vi "ScopeDAQ.vi"() -> ()   [LabVIEW 2021]
uses:
  <instrlib>/Tektronix TDS 200 1000 2000 Series/Public/Configure/Configure Trigger (Edge).vi
  <instrlib>/Tektronix TDS 200 1000 2000 Series/Tektronix TDS 200 1000 2000 Series.lvlib
panel:
  in  "Signal Source (Channel)":u16(ring) items=["Channel 1", "Channel 2", "Channel 3", "Channel 4", "Math", "Reference A", "Reference B", "Reference C", "Reference D"]
  in  "Position (0.0 s)":dbl
  out "Waveform Graph":waveform(dbl)(graph)={"t0"=timestamp(-2.500000000016378e-06 s since 1904-01-01), "dt"=2e-09, "Y"=array[2500 elements]}
  in  "Trigger Level (V)":dbl=-0.368
  in  "Vertical Range (V/div)":dbl=0.5
  in  "Timebase (s/div)":dbl=5e-07
  in  "Vertical Coupling":i32(ring) items=["AC", "DC", "Ground"]
  in  "Serial Configuration":T1={"Baud Rate"=19200, "Parity"=0, "Stop Bits"=10, "Flow Control"=2} {"Flow Control" items=["None", "XON/XOFF", "RTS/CTS", "XON/XOFF & RTS/CTS", "DTR/DSR", "XON/XOFF & DTR/DSR"]; "Stop Bits" items=["1.0"=10, "1.5"=15, "2.0"=20]; "Parity" items=["None", "Odd", "Even", "Mark", "Space"]; "Baud Rate" items=["300"=300, "600"=600, "1200"=1200, "2400"=2400, "4800"=4800, "9600"=9600, "19200"=19200]}
  in  "Trigger Source (Channel)":u16(ring) items=["Channel 1", "Channel 2", "Channel 3", "Channel 4", "Math", "Reference A", "Reference B", "Reference C", "Reference D"]
  in  "stop":bool
  in  "Probe Attenuation":dbl=1.0
  in  "VISA resource name":refnum<visa-resource-name>="USB0::0x0699::0x0369::C057527::INSTR"
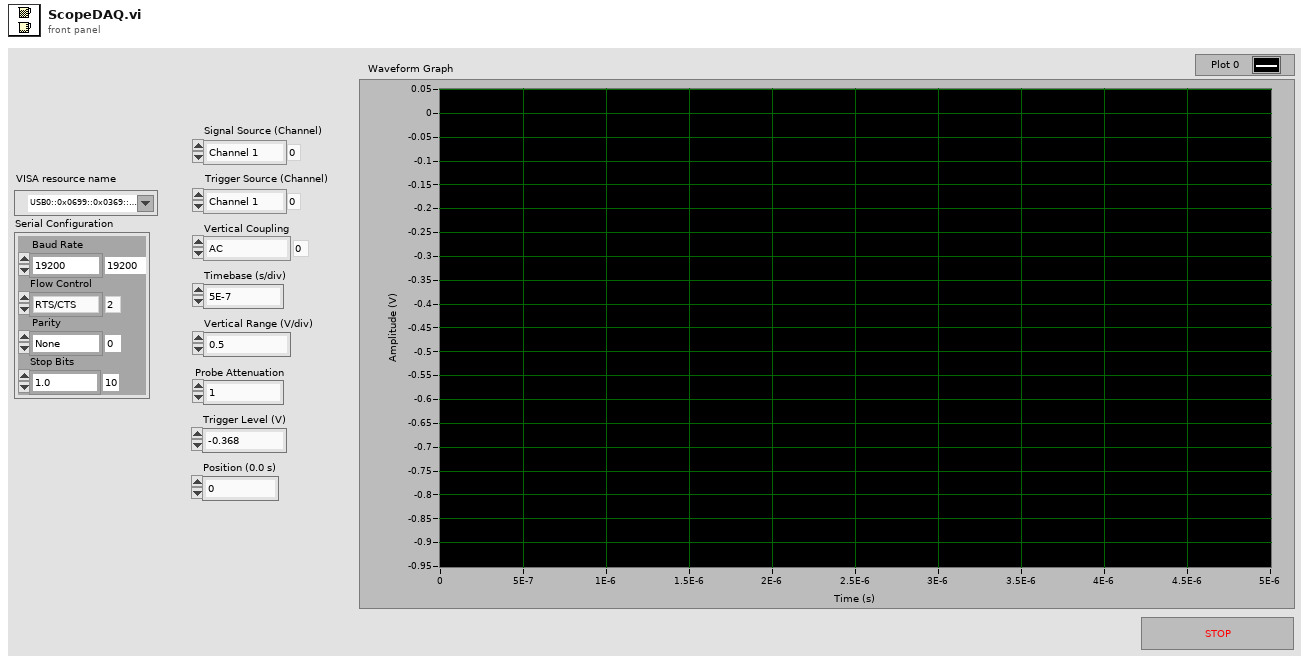
[diagram p1: front panel]
types:
  T1 = cluster{"Baud Rate":u32, "Parity":u16, "Stop Bits":u16, "Flow Control":u16}
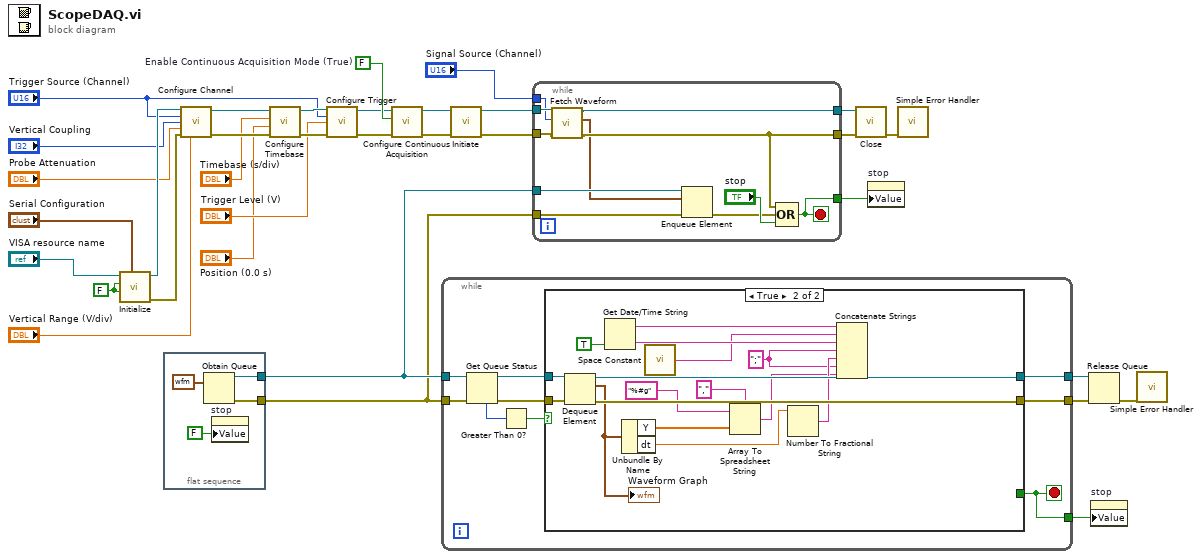
[diagram p0: block diagram]
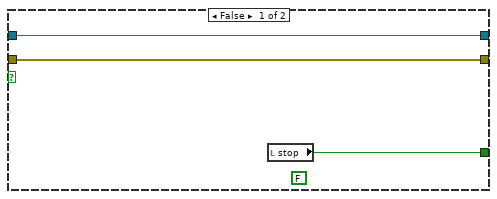
[diagram p2: hidden frame]
diagram:
  w10 = FALSE  # Enable Continuous Acquisition Mode (True)
  w33 = FALSE ("ID Query? (T: Yes)")
  n1 = call <instrlib>:"Initialize.vi"("Serial Configuration"="Serial Configuration", "Reset? (T: Yes)"=w33, "ID Query? (T: Yes)"=w33, "VISA resource name"="VISA resource name") -> ("error out"=w25:errorcluster, "VISA resource name out"=w26:refnum<visa-resource-name>)  [unwired: 6 in]
  n2 = flat-sequence {
    tunnel: [w37] -> w19
    tunnel: [w38] -> w20
    frame #0 {
      n3 = Obtain Queue(element data type=waveform(dbl) {"t0"=timestamp(0 s since 1904-01-01), "dt"=1.0, "Y"=[]} ("Waveform Data")) -> (queue out=w38:refnum<queue>, error out=w37:errorcluster)  [unwired: 4 in, 1 out]
      n4 = property on="stop" class="Bool (strict)"("Value"=FALSE ("stop")) -> ()  [unwired: 2 in, 2 out]
    }
  }
  n5 = call <instrlib>:"Configure Channel.vi"("VISA resource name"=w26, "Channel (0: Channel 1)"="Trigger Source (Channel)", "Vertical Coupling (1: DC)"="Vertical Coupling", "Probe Attenuation (10: 10X)"="Probe Attenuation", "error in (no error)"=w25, "Vertical Range (10.0 V/div)"="Vertical Range (V/div)") -> ("VISA resource name out"=w28:refnum<visa-resource-name>, "error out"=w27:errorcluster)  [unwired: 8 in]
  n6 = call <instrlib>:"Configure Timebase.vi"("error in (no error)"=w27, "Position (0.0 s)"="Position (0.0 s)", "Timebase (0.0005 s)"="Timebase (s/div)", "VISA resource name"=w28) -> ("error out"=w14:errorcluster, "VISA resource name out"=w15:refnum<visa-resource-name>)  [unwired: 6 in]
  n7 = call-poly <instrlib>:"Configure Trigger.vi"("VISA resource name"=w15, "Trigger Source (0: Channel 1)"="Trigger Source (Channel)", "Trigger Level (0.0 V)"="Trigger Level (V)", "error in (no error)"=w14) -> ("VISA resource name out"=w7:refnum<visa-resource-name>, "error out"=w6:errorcluster)  [unwired: 10 in]
  n8 = call <instrlib>:"Configure Continuous Acquisition.vi"("error in (no error)"=w6, "Enable Continuous Acquisition Mode (True)"=w10, "VISA resource name"=w7) -> ("error out"=w9:errorcluster, "VISA resource name out"=w8:refnum<visa-resource-name>)  [unwired: 7 out]
  n9 = while {
    tunnel: w20 -> [w47]
    tunnel: w19 -> [w46]
    tunnel: [w42] -> w18
    tunnel: [w41] -> w17
    tunnel: [w40] -> w11
    stop <- w40 stop-if-true
    n10 = Get Queue Status(queue=w47, error in (no error)=w46) -> (queue out=w45:refnum<queue>, error out=w44:errorcluster, # elements in queue=w43:i32)  [unwired: 1 in, 5 out]
    n11 = Greater Than 0?(x=w43) -> (x > 0?=w39:bool)
    n12 = case shown="True" w39 {
      tunnel: w45 -> [w50 w62]
      tunnel: w44 -> [w49 w61]
      tunnel: [w50 w60] -> w42
      tunnel: [w49 w66] -> w41
      tunnel: [w48 _] -> w40
      frame False {
        (unwired) FALSE
        n13 = local read "stop"() -> (w48:bool)
      }
      frame True {
        w54 = ";" ("string")
        n14 = Dequeue Element(queue=w62, error in (no error)=w61) -> (queue out=w60:refnum<queue>, element=w53:waveform(dbl), error out=w66:errorcluster)  [unwired: 1 in, 1 out]
        "Waveform Graph" <- w53
        n15 = Get Date/Time String(want seconds? (F)=TRUE) -> (date string=w64:string, time string=w63:string)  [unwired: 2 in]
        n16 = Unbundle By Name(w53) -> ("Y"=w51:dbl[], "dt"=w58:dbl)
        n17 = call <vilib>:"Space Constant.vi"() -> ("String"=w55:string)
        n18 = Array To Spreadsheet String(delimiter (Tab)=",", array=w51, 3:"%#g" ("format string")) -> (spreadsheet string=w56:string)
        n19 = Number To Fractional String(number=w58) -> (F-format string=w57:string)  [unwired: 3 in]
        n20 = Concatenate Strings(w64, w55, w63, w54, w57, w54, w56) -> ()  [unwired: 1 out]
      }
    }
  }
  n21 = call <instrlib>:"Initiate.vi"("error in (no error)"=w9, "VISA resource name"=w8) -> ("error out"=w4:errorcluster, "VISA resource name out"=w5:refnum<visa-resource-name>)  [unwired: 8 out]
  n22 = while {
    tunnel: [w70] -> w30
    tunnel: [w69] -> w29
    tunnel: w20 -> [w77]
    tunnel: w19 -> [w76]
    tunnel: w5 -> [w72]
    tunnel: w4 -> [w71]
    tunnel: [w74] -> w12
    tunnel: "Signal Source (Channel)" -> [w68]
    stop <- w74 stop-if-true
    n23 = call <instrlib>:"Fetch Waveform.vi"("error in (no error)"=w71, "Source (0: Channel 1)"=w68, "VISA resource name"=w72) -> ("error out"=w69:errorcluster, "Waveform Data"=w67:waveform(dbl), "VISA resource name out"=w70:refnum<visa-resource-name>)  [unwired: 1 in, 5 out]
    n24 = Enqueue Element(queue=w77, element=w67, error in (no error)=w76) -> (error out=w73:errorcluster)  [unwired: 1 in, 2 out]
    n25 = Compound Arithmetic op=OR(w69, w73, "stop") -> (w74:bool)
  }
  n26 = call <instrlib>:"Close.vi"("error in (no error)"=w29, "VISA resource name"=w30) -> ("error out"=w31:errorcluster)  [unwired: 9 in]
  n27 = property on="stop" class="Bool (strict)"("Value"=w12) -> ()  [unwired: 2 in, 2 out]
  n28 = call <vilib>:"Simple Error Handler.vi"("error in (no error)"=w31) -> ()  [unwired: 1 in, 8 out]
  n29 = Release Queue(queue=w18, error in (no error)=w17) -> (error out=w16:errorcluster)  [unwired: 1 in, 2 out]
  n30 = property on="stop" class="Bool (strict)"("Value"=w11) -> ()  [unwired: 2 in, 2 out]
  n31 = call <vilib>:"Simple Error Handler.vi"("error in (no error)"=w16) -> ()  [unwired: 1 in, 8 out]
